vi "tranform_gen.vi"(0 "Array":cluster{"Coords":T2, dbl[]}[](array[cluster])) -> (1 "transformation matrix":T1, 2 "offset":dbl[](array[numeric]))   [LabVIEW 2017]
uses:
  <vilib>/Utility/miscctls.llb/LVPoint32TypeDef.ctl
  <vilib>/Analysis/Matrix/Datatypes/RealMatrix.ctl
  <vilib>/Analysis/Matrix/NI_Matrix.lvlib
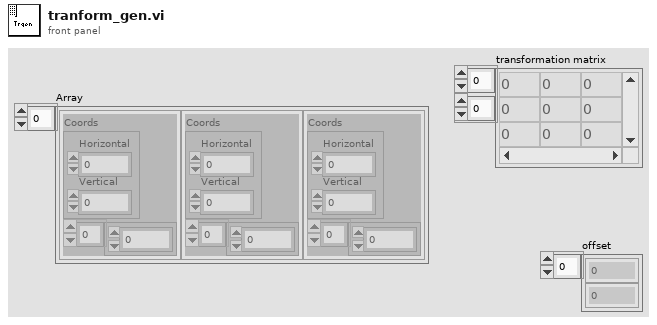
[diagram p1: front panel]
types:
  T1 = typedef "NI_Matrix.lvlib/RealMatrix.ctl" = dbl[][]
  T2 = typedef "LVPoint32TypeDef.ctl" = cluster{"Horizontal":i32, "Vertical":i32}
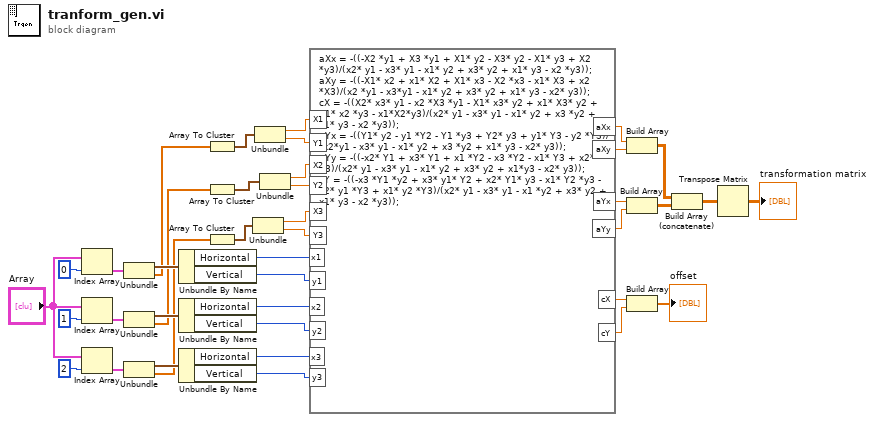
[diagram p0: block diagram]
diagram:
  n1 = Index Array(array="Array", index=0) -> (element=w25:cluster{"Coords":T2, dbl[]})
  n2 = Index Array(array="Array", index=1) -> (element=w22:cluster{"Coords":T2, dbl[]})
  n3 = Index Array(array="Array", index=2) -> (element=w19:cluster{"Coords":T2, dbl[]})
  n4 = Unbundle(w25) -> ("Coords"=w24:T2, w23:dbl[])
  n5 = Unbundle(w22) -> ("Coords"=w21:T2, w20:dbl[])
  n6 = Unbundle(w19) -> ("Coords"=w18:T2, w17:dbl[])
  n7 = Unbundle By Name(w24) -> ("Horizontal"=w12:i32, "Vertical"=w11:i32)
  n8 = Unbundle By Name(w21) -> ("Horizontal"=w10:i32, "Vertical"=w9:i32)
  n9 = Unbundle By Name(w18) -> ("Horizontal"=w8:i32, "Vertical"=w7:i32)
  n10 = Array To Cluster(array=w23) -> (cluster=w13:cluster{"[0]":dbl, "[1]":dbl})
  n11 = Array To Cluster(array=w20) -> (cluster=w14:cluster{"[0]":dbl, "[1]":dbl})
  n12 = Array To Cluster(array=w17) -> (cluster=w15:cluster{"[0]":dbl, "[1]":dbl})
  n13 = Unbundle(w15) -> ("[0]"=w2:dbl, "[1]"=w1:dbl)
  n14 = Unbundle(w13) -> ("[0]"=w6:dbl, "[1]"=w5:dbl)
  n15 = Unbundle(w14) -> ("[0]"=w4:dbl, "[1]"=w3:dbl)
  n16 = formula code="aXx = -((-X2 *y1 + X3 *y1 + X1* y2 - X3* y2 - X1* y3 + X2 *y3)/(x2* y1 - x3* y1 - x1* y2 + x3* y2 + x1* y3 - x2 *y3)); \naXy = -((-X1* x2 + x1* X2 + X1* x3 - X2 *x3 - x1* X3 + x2 *X3)/(x2 *y1 - x3*y1 - x1* y2 + x3* y2 + x1* y3 - x2* y3)); \ncX = -((X2* x3* y1 - x2 *X3 *y1 - X1* x3* y2 + x1* X3* y2 + X1* x2 *y3 - x1*X2*y3)/(x2* y1 - x3* y1 - x1* y2 + x3 *y2 + x1* y3 - x2 *y3)); \naYx = -((Y1* y2 - y1 *Y2 - Y1 *y3 + Y2* y3 + y1* Y3 - y2 *Y3)/(x2*y1 - x3* y1 - x1* y2 + x3 *y2 + x1* y3 - x2* y3)); \naYy = -((-x2* Y1 + x3* Y1 + x1 *Y2 - x3 *Y2 - x1* Y3 + x2* Y3)/(x2* y1 - x3* y1 - x1* y2 + x3* y2 + x1*y3 - x2* y3)); \ncY = -((-x3 *Y1 *y2 + x3* y1* Y2 + x2* Y1* y3 - x1* Y2 *y3 - x2* y1 *Y3 + x1* y2 *Y3)/(x2* y1 - x3* y1 - x1 *y2 + x3* y2 + x1* y3 - x2 *y3));"("X1"=w6, "Y1"=w5, "X3"=w2, "Y3"=w1, "x2"=w10, "y2"=w9, "x3"=w8, "X2"=w4, "Y2"=w3, "x1"=w12, "y1"=w11, "y3"=w7) -> ("aXx"=w37:dbl, "aXy"=w36:dbl, "cX"=w33:dbl, "aYx"=w35:dbl, "aYy"=w34:dbl, "cY"=w32:dbl)
  n17 = Build Array(w37, w36) -> (w38:T1)
  n18 = Build Array(w35, w34) -> (w39:T1)
  n19 = Build Array(w33, w32) -> (→"offset":dbl[])
  n20 = Build Array (concatenate)(w38, w39) -> (w31:T1)
  n21 = Transpose Matrix(1:w31) -> (0:→"transformation matrix":T1)
